vi "vi in lib.vi"(8 "Numeric":dbl=25.0) -> (0 "x+y":dbl)   [LabVIEW 2021, in "lib.lvlib"]
uses:
  lib.lvlib
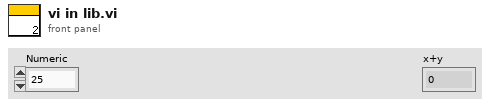
[diagram p1: front panel]
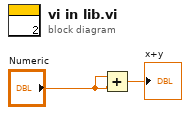
[diagram p0: block diagram]
diagram:
  n1 = Add(x="Numeric", y="Numeric") -> (x+y=→"x+y":dbl)
